vi "Restore Panel Data.vi"(8 "error in (no error)":errorcluster, 10 "EditPanel API in":refnum<class "EditPanel API.lvclass">, 11 "Console Reply In":refnum<class "Console Reply.lvclass">) -> (0 "error out":errorcluster, 2 "EditPanel API out":refnum<class "EditPanel API.lvclass">, 3 "Console Reply Out":refnum<class "Console Reply.lvclass">)   [LabVIEW 2015, in "EditPanel API.lvlib" / "Console Reply.lvclass"]
uses:
  Console Reply.lvclass
  EditPanel_class/EditPanel API.lvclass
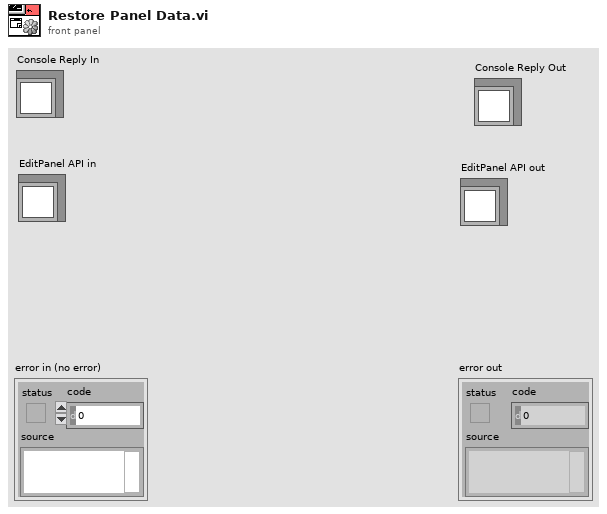
[diagram p1: front panel]
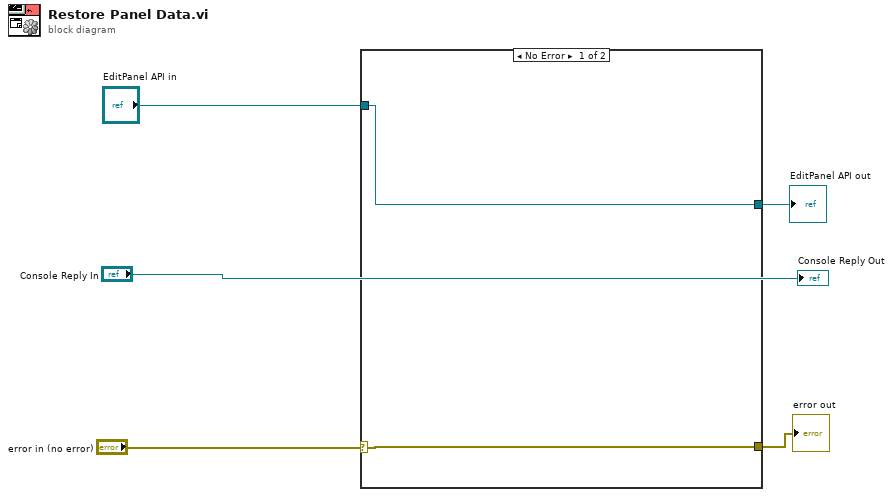
[diagram p0: block diagram]
diagram:
  n1 = case shown="No Error" "error in (no error)" {
    selector: "error in (no error)" -> [w6 w8]
    tunnel: "EditPanel API in" -> [w7 w9]
    tunnel: [w6 w8] -> w4
    tunnel: [w7 w9] -> w3
    frame No Error {
    }
    frame Error {
    }
  }
  "error out" <- w4
  "EditPanel API out" <- w3
  "Console Reply Out" <- "Console Reply In"
